vi "切换出图模式.vi"(8 "error in":errorcluster, 10 "模式":u8) -> (0 "error out":errorcluster, 2 "return":i32)   [LabVIEW 2016]
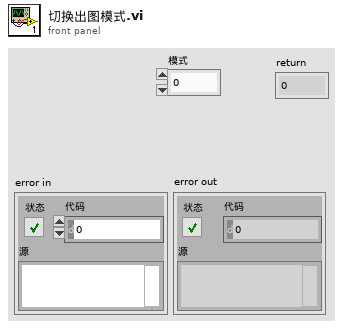
[diagram p1: front panel]
types:
  T1 = cluster{"byCmdType":u8, "bySubCmd":u8, "byPara":u8, "byAddr_h":u8, "byAddr_l":u8, "byAddr_ll":u8, "byLen_h":u8, "byLen_l":u8}
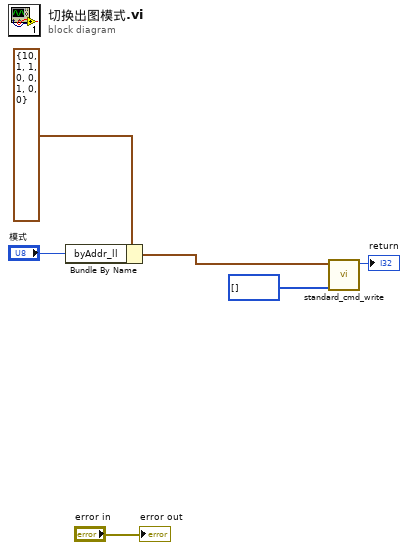
[diagram p0: block diagram]
diagram:
  n1 = Bundle By Name(cluster=T1 {"byCmdType"=10, "bySubCmd"=1, "byPara"=1, "byAddr_h"=0, "byAddr_l"=0, "byAddr_ll"=1, "byLen_h"=0, "byLen_l"=0} ("cmd_std_header_t"), "byAddr_ll"="模式") -> (w2:T1)
  n2 = call "standard_cmd_write.vi"("data"=u8[] [], "cmd_std_header_t"=w2) -> ("return"=→"return":i32)  [unwired: 9 in]
  "error out" <- "error in"
